vi "rethinkdb_msg_response.vi"(8 "error in (no error)":errorcluster, 11 "response":string) -> (0 "error out":errorcluster, 3 "elements":T1[](array[typedef]))   [LabVIEW 2017]
uses:
  json/json_element.ctl
  json/json_element_type.ctl
  8958eac0-6979-464f-ae0a-bdee0e6a396b.vi
  b7d8fced-4970-4fca-bbc6-92f1d5f3337a.vi
  a3bdcb10-d031-440d-baf2-ef98e914bb66.vi
  json/json_parse_value.vi
  json/json_resolve_key.vi
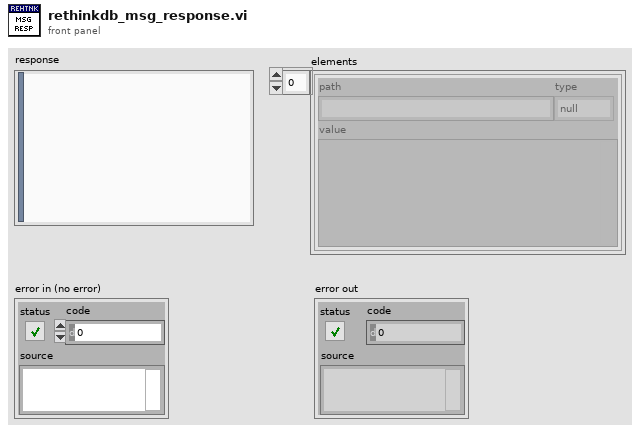
[diagram p1: front panel]
types:
  T1 = typedef "json_element.ctl" = cluster{"path":string, "type":T2, "value":variant}
  T2 = typedef "json_element_type.ctl" = enum8{"null", "bool", "int", "uint", "float", "string", "array", "object"}
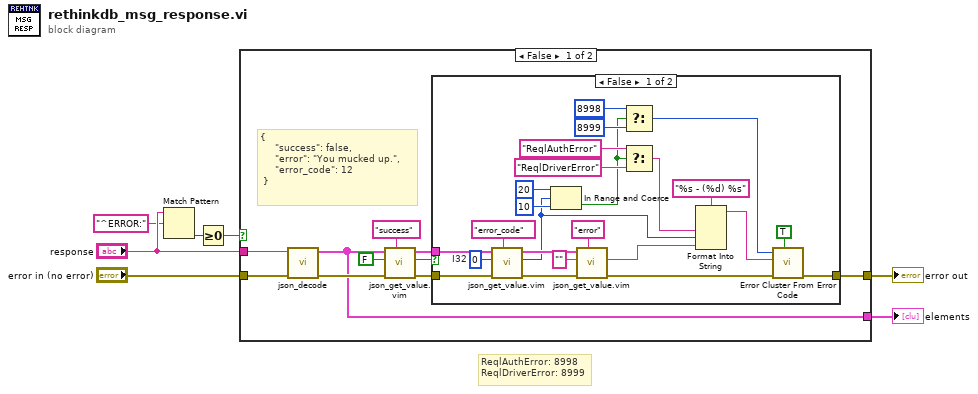
[diagram p0: block diagram]
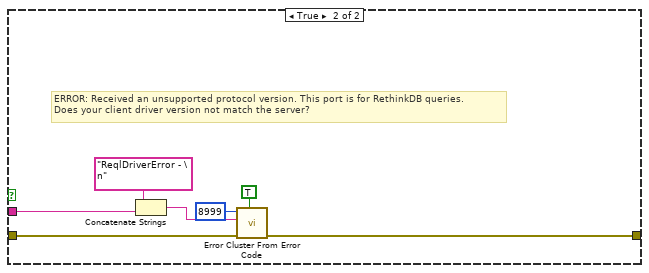
[diagram p3: hidden frame]
diagram:
  # "ReqlAuthError: 8998\nReqlDriverError: 8999"
  n1 = Match Pattern(string="response", regular expression="^ERROR:") -> (offset past match=w3:i32)  [unwired: 1 in, 3 out]
  n2 = Greater Or Equal To 0?(x=w3) -> (x >= 0?=w2:bool)
  n3 = case shown="False" w2 {
    tunnel: "error in (no error)" -> [w17 w46]
    tunnel: "response" -> [w10 w44]
    tunnel: [w9 w45] -> w4
    tunnel: [w8 _] -> w1
    frame False {
      # "{\n     \"success\": false,\n     \"error\": \"You mucked up.\",\n     \"error_code\": 12\n }"
      n4 = call "json_decode.vi"("error in (no error)"=w17, "json"=w10) -> ("error out"=w16:errorcluster, "elements"=w8:T1[])  [unwired: 8 in]
      n5 = call "json_get_value.vim"("key"="success", "error in (no error)"=w16, "default"=FALSE, "elements in"=w8) -> ("error out"=w12:errorcluster, "value"=w13:bool, "elements out"=w11:T1[])  [unwired: 4 in, 1 out]
      n6 = case shown="False" w13 {
        tunnel: w12 -> [w40 w42]
        tunnel: w11 -> [w39 _]
        tunnel: [w29 w42] -> w9
        frame False {
          w38 = 0  # I32
          n7 = call "json_get_value.vim"("key"="error_code", "error in (no error)"=w40, "default"=w38, "elements in"=w39) -> ("error out"=w35:errorcluster, "value"=w27:i32, "elements out"=w36:T1[])  [unwired: 4 in, 1 out]
          n8 = In Range and Coerce(upper limit=20, x=w27, lower limit=10) -> (In Range?=w19:bool)  [unwired: 1 out]
          n9 = call "json_get_value.vim"("key"="error", "error in (no error)"=w35, "default"="", "elements in"=w36) -> ("error out"=w30:errorcluster, "value"=w28:string)  [unwired: 4 in, 2 out]
          n10 = Select(t=8998 ("error code (0)"), s=w19, f=8999 ("error code (0)")) -> (s? t:f=w18:i32)
          n11 = Select(t="ReqlAuthError", s=w19, f="ReqlDriverError") -> (s? t:f=w22:string)
          n12 = Format Into String(format string="%s - (%d) %s" ("error message (\"\")"), w22, w27, w28) -> (resulting string=w23:string)  [unwired: 2 in, 1 out]
          n13 = call <vilib>:"Error Cluster From Error Code.vi"("show call chain? (False)"=TRUE, "error in (no error)"=w30, "error message (\"\")"=w23, "error code (0)"=w18) -> ("error out"=w29:errorcluster)  [unwired: 5 in]
        }
        frame True {
        }
      }
    }
    frame True {
      # "ERROR: Received an unsupported protocol version. This port is for RethinkDB queries. \nDoes your client driver version not match the server?"
      n14 = Concatenate Strings("ReqlDriverError - \n" ("error message (\"\")"), w44) -> (w43:string)
      n15 = call <vilib>:"Error Cluster From Error Code.vi"("show call chain? (False)"=TRUE, "error in (no error)"=w46, "error message (\"\")"=w43, "error code (0)"=8999) -> ("error out"=w45:errorcluster)  [unwired: 5 in]
    }
  }
  "error out" <- w4
  "elements" <- w1
